vi "Get Scene Item Enabled.vi"(8 "error in (no error)":errorcluster, 9 "Scene Item ID":i32, 10 "Scene Name":string, 11 "OBS in":refnum<class "OBS.lvclass">) -> (0 "error out":errorcluster, 2 "Enabled":bool, 3 "OBS out":refnum<class "OBS.lvclass">)   [LabVIEW 2022 SP3, in "obs-websocket-lv.lvlib" / "OBS.lvclass"]
uses:
  OBS.lvclass
  OBS.lvclass/OBS.ctl
  GetSceneItemEnabled/GetSceneItemEnabled.lvclass
  RGetSceneItemEnabled/RGetSceneItemEnabled.lvclass
  C:/dev/illuminatedg/obs-websocket-lv/obs-websocket-lv/Response/Response.lvclass
  C:/dev/illuminatedg/obs-websocket-lv/obs-websocket-lv/Server Message/Server Message.lvclass
  C:/dev/illuminatedg/obs-websocket-lv/obs-websocket-lv/Message/Message.lvclass
  C:/dev/illuminatedg/obs-websocket-lv/obs-websocket-lv/RGetSceneItemEnabled/RGetSceneItemEnabled.lvclass
  C:/dev/illuminatedg/obs-websocket-lv/obs-websocket-lv/Request/Request.lvclass
  C:/dev/illuminatedg/obs-websocket-lv/obs-websocket-lv/Client Message/Client Message.lvclass
  C:/dev/illuminatedg/obs-websocket-lv/obs-websocket-lv/GetSceneItemEnabled/GetSceneItemEnabled.lvclass
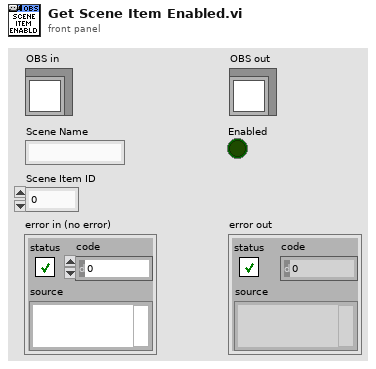
[diagram p1: front panel]
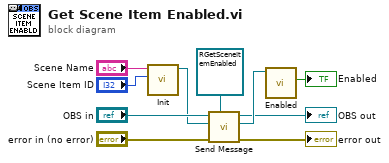
[diagram p0: block diagram]
diagram:
  n1 = call "Init.vi"("Scene Item ID"="Scene Item ID", "Scene Name"="Scene Name") -> ("GetSceneItemEnabled out"=w6:refnum<class "GetSceneItemEnabled.lvclass">)  [unwired: 8 in, 1 out]
  n2 = call "Send Message.vi"("Response Type (None)"=refnum<class "RGetSceneItemEnabled.lvclass"> refnum ("obs-websocket-lv.lvlib:RGetSceneItemEnabled.lvclass"), "error in (no error)"="error in (no error)", "Client Message"=w6, "OBS in"="OBS in") -> ("error out"=→"error out":errorcluster, "Response"=w4:refnum<class "RGetSceneItemEnabled.lvclass">, "OBS out"=→"OBS out":refnum<class "OBS.lvclass">)  [unwired: 4 in, 1 out]
  n3 = call "Enabled.vi"("RGetSceneItemEnabled in"=w4) -> ("Enabled"=→"Enabled":bool)  [unwired: 8 in, 2 out]
